vi "SetStageBusy_Status_MotorController.vi"(8 "error in (no error)":errorcluster, 10 "Stage Busy?":bool, 11 "Motor Controller in":refnum<class "Motor Controller.lvclass">) -> (0 "error out":errorcluster, 3 "Motor Controller out":refnum<class "Motor Controller.lvclass">)   [LabVIEW 2022 SP3, in "Motor Controller.lvclass"]
uses:
  Motor Controller.lvclass
  Motor Controller.lvclass/Motor Controller.ctl
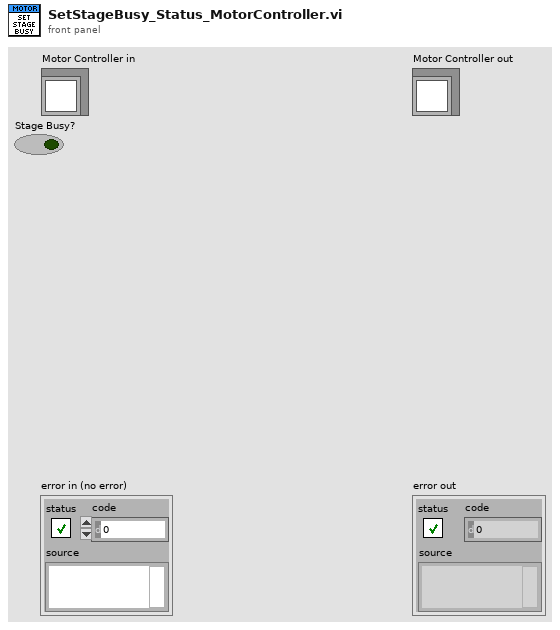
[diagram p1: front panel]
types:
  T1 = typedef "Motor Controller.lvclass/Private Data.ctl" = cluster{"UserEvents":T2, "All Dependencies":cluster{"Class References":refnum<class>[], "Class Names":string[]}, "Status":T3}
  T2 = typedef "Motor Controller.lvclass/UserEvents.ctl" = cluster{"API Incoming Event":refnum<user-event>, "API Executed Event":refnum<user-event>, "API Return Event":refnum<user-event>, "Status Changed Event":refnum<user-event>, "StopEvent":refnum<user-event>}
  T3 = typedef "Motor Controller.lvclass/Status.ctl" = cluster{"Motor Controller Config Data":T4, "Motor Controller Data":cluster{"Enabled?":bool}, "Stage Move":T5, "Stage Busy?":bool}
  T4 = typedef "Motor Controller.lvclass/Motor Controller Config Data.ctl" = cluster{"Motor IP Addresss":string, "Current Position":i32, "Pulse_Per_mm":i32, "PrePrint":dbl[], "Load Position_mm":i32, "Laminate Position_mm":i32}
  T5 = typedef "Motor Controller.lvclass/Stage Move Data.ctl" = cluster{"Current Step":string, "Move Data":T6[]}
  T6 = typedef "Motor Controller.lvclass/Batch Index Speed Data.ctl" = cluster{"Batch & Cycle":string, "Move":cluster{"Index_mm":i32, "Speed_mm_s":i32}, "Status":T7}
  T7 = typedef "Motor Controller.lvclass/Move Status.ctl" = enum16{"Pending", "In Progress", "Completed"}
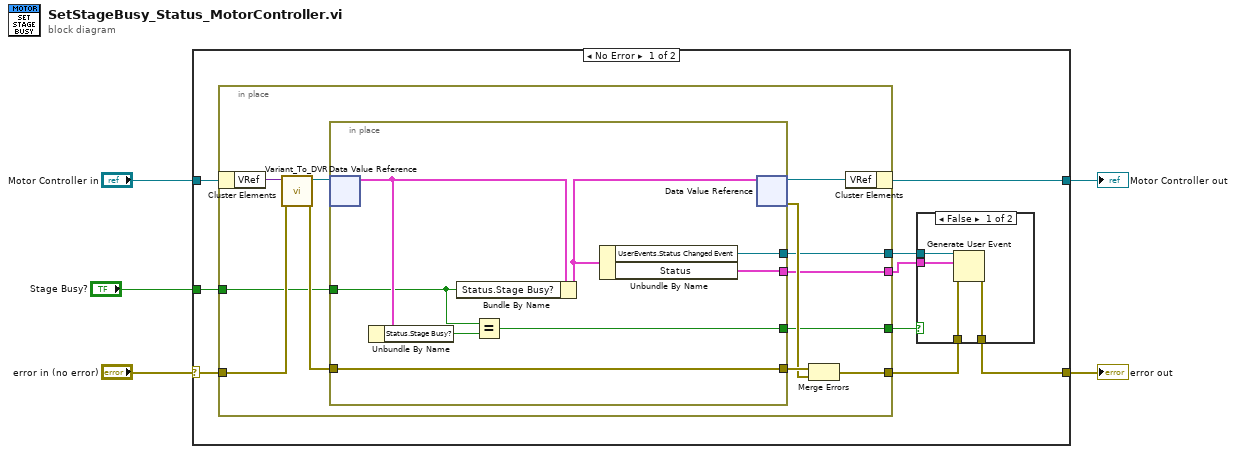
[diagram p0: block diagram]
diagram:
  n1 = case shown="No Error" "error in (no error)" {
    selector: "error in (no error)" -> [w12 w41]
    tunnel: [w9 w41] -> w2
    tunnel: [w14 w40] -> w3
    tunnel: "Motor Controller in" -> [w13 w40]
    tunnel: "Stage Busy?" -> [w7 _]
    frame No Error {
      n2 = in-place {
        in-place-border: w12 -> [w29]
        in-place-border: [w25] -> w10
        in-place-border: [w23] -> w11
        in-place-border: [w22] -> w8
        in-place-border: w7 -> [w21]
        in-place-border: [w20] -> w6
        n3 = in-place-cluster #1(w13) -> ("VRef"=w31:variant)
        n4 = call "Variant_To_DVR.vi"("error in (no error)"=w29, "Variant"=w31) -> ("error out"=w28:errorcluster, "DVR"=w30:refnum<data-value>)  [unwired: 8 in]
        n5 = in-place {
          in-place-border: w28 -> [w39]
          in-place-border: [w39] -> w27
          in-place-border: [w37] -> w23
          in-place-border: [w36] -> w22
          in-place-border: w21 -> [w33]
          in-place-border: [w32] -> w20
          n6 = in-place-dvr #2(w30) -> (w35:T1)  [unwired: 1 out]
          n7 = Unbundle By Name(w35) -> ("Status.Stage Busy?"=w34:bool)
          n8 = Bundle By Name(cluster=w35, "Status.Stage Busy?"=w33) -> (w38:T1)
          n9 = Equal?(x=w33, y=w34) -> (x = y?=w32:bool)
          n10 = Unbundle By Name(w38) -> ("UserEvents.Status Changed Event"=w37:refnum<user-event>, "Status"=w36:T3)
          n11 = in-place-dvr #2(w38) -> (w24:refnum<data-value>, w26:errorcluster)
        }
        n12 = Merge Errors(w27, w26) -> (w25:errorcluster)
        n13 = in-place-cluster #1("VRef"=w24) -> (w14:refnum<class "Motor Controller.lvclass">)
      }
      n14 = case shown="False" w6 {
        tunnel: w11 -> [w18 _]
        tunnel: w10 -> [w17 w19]
        tunnel: [w16 w19] -> w9
        tunnel: w8 -> [w15 _]
        frame False {
          n15 = Generate User Event(user event=w18, event data cluster=w15, error in=w17) -> (error out=w16:errorcluster)  [unwired: 1 in, 1 out]
        }
        frame True {
        }
      }
    }
    frame Error {
    }
  }
  "error out" <- w2
  "Motor Controller out" <- w3
